vi "Find.vi"(8 "Error In":errorcluster, 10 "Key":string, 11 "Context In":refnum<class "Context.lvclass">) -> (0 "Error Out":errorcluster, 1 "Found?":bool, 2 "Datum":refnum<class "Abstract.lvclass">, 3 "Context Out":refnum<class "Context.lvclass">)   [LabVIEW 2018, in "Toolkit.lvlib" / "Data.lvlib" / "Context.lvclass"]
uses:
  Context.lvclass
  Abstract/Abstract.lvclass
  Context.lvclass/Context.ctl
  Null/Null.lvclass
  D:/Users/cfield/Code/Field R&D Services/Mustache/trunk/src/Toolkit/Data/Abstract/Abstract.lvclass
  Map/Map.lvclass
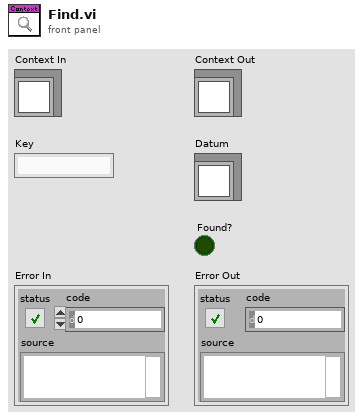
[diagram p1: front panel]
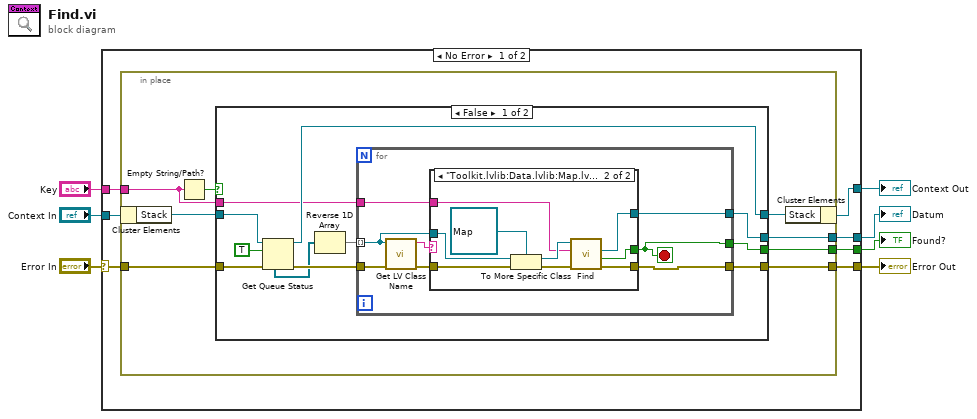
[diagram p0: block diagram]
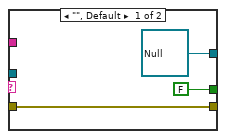
[diagram p2: hidden frame]
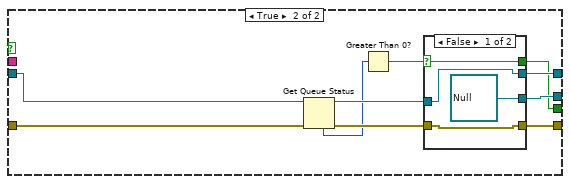
[diagram p3: hidden frame]
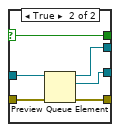
[diagram p4: hidden frame]
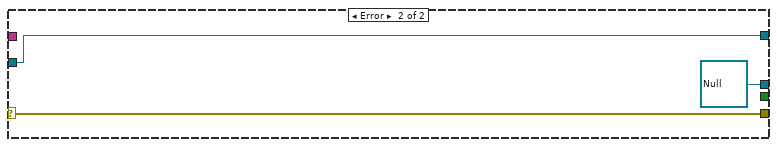
[diagram p5: hidden frame]
diagram:
  n1 = case shown="No Error" "Error In" {
    selector: "Error In" -> [w11 w75]
    tunnel: [w14 refnum<class "Null.lvclass"> refnum ("Toolkit.lvlib:Data.lvlib:Null.lvclass")] -> w7
    tunnel: [w13 w75] -> w6
    tunnel: [w12 _] -> w5
    tunnel: "Context In" -> [w10 w76]
    tunnel: [w9 w76] -> w2
    tunnel: "Key" -> [w8 _]
    frame No Error {
      n2 = in-place {
        in-place-border: [w22] -> w14
        in-place-border: [w21] -> w13
        in-place-border: [w20] -> w12
        in-place-border: w11 -> [w19]
        in-place-border: w8 -> [w16]
        n3 = in-place-cluster #1(w10) -> ("Stack"=w18:refnum<queue>)
        n4 = Empty String/Path?(string/path=w16) -> (empty?=w15:bool)
        n5 = case shown="False" w15 {
          tunnel: [w33 w62] -> w22
          tunnel: [w32 w54] -> w21
          tunnel: [w27 w55] -> w20
          tunnel: w19 -> [w26 w58]
          tunnel: w18 -> [w25 w61]
          tunnel: [w24 w63] -> w17
          tunnel: w16 -> [w23 _]
          frame False {
            n6 = Get Queue Status(queue=w25, return elements? (F)=TRUE, error in (no error)=w26) -> (queue out=w24:refnum<queue>, error out=w31:errorcluster, elements=w29:refnum<class "Abstract.lvclass">[])  [unwired: 5 out]
            n7 = Reverse 1D Array(array=w29) -> (reversed array=w30:refnum<class "Abstract.lvclass">[])
            n8 = for {
              tunnel: w30 -> [w38] mode=indexing
              tunnel: w23 -> [w37]
              tunnel: w31 -> [w41]
              tunnel: [w36] -> w32
              tunnel: [w35] -> w33
              tunnel: [w34] -> w27
              stop <- w34 stop-if-true
              n9 = call <vilib>:"Get LV Class Name.vi"("error in (no error)"=w41, "object"=w38) -> ("error out"=w39:errorcluster, "class name"=w40:string)  [unwired: 8 in]
              n10 = case shown="\"Toolkit.lvlib:Data.lvlib:Map.lvclass\"" w40 {
                tunnel: w39 -> [w43 w53]
                tunnel: w38 -> [_ w52]
                tunnel: w37 -> [_ w48]
                tunnel: [w43 w47] -> w36
                tunnel: [FALSE ("Found?") w45] -> w34
                tunnel: [refnum<class "Null.lvclass"> refnum ("Toolkit.lvlib:Data.lvlib:Null.lvclass") w46] -> w35
                frame "", Default {
                }
                frame "Toolkit.lvlib:Data.lvlib:Map.lvclass" {
                  n11 = To More Specific Class(target class=refnum<class "Map.lvclass"> refnum ("Toolkit.lvlib:Data.lvlib:Map.lvclass"), reference=w52, error in=w53) -> (specific class reference=w49:refnum<class "Map.lvclass">, error out=w50:errorcluster)
                  n12 = call "Find.vi"("Error In"=w50, "Key"=w48, "Map In"=w49) -> ("Error Out"=w47:errorcluster, "Found?"=w45:bool, "Value"=w46:refnum<class "Abstract.lvclass">)  [unwired: 5 in, 1 out]
                }
              }
            }
          }
          frame True {
            n13 = Get Queue Status(queue=w61, error in (no error)=w58) -> (queue out=w60:refnum<queue>, error out=w59:errorcluster, # elements in queue=w57:i32)  [unwired: 1 in, 5 out]
            n14 = Greater Than 0?(x=w57) -> (x > 0?=w56:bool)
            n15 = case shown="False" w56 {
              selector: w56 -> [w66 w68]
              tunnel: [w67 w73] -> w63
              tunnel: [refnum<class "Null.lvclass"> refnum ("Toolkit.lvlib:Data.lvlib:Null.lvclass") w72] -> w62
              tunnel: w60 -> [w67 w71]
              tunnel: w59 -> [w65 w70]
              tunnel: [w66 w68] -> w55
              tunnel: [w65 w69] -> w54
              frame False {
              }
              frame True {
                n16 = Preview Queue Element(queue=w71, error in (no error)=w70) -> (queue out=w73:refnum<queue>, element=w72:refnum<class "Abstract.lvclass">, error out=w69:errorcluster)  [unwired: 1 in, 1 out]
              }
            }
          }
        }
        n17 = in-place-cluster #1("Stack"=w17) -> (w9:refnum<class "Context.lvclass">)
      }
    }
    frame Error {
    }
  }
  "Datum" <- w7
  "Error Out" <- w6
  "Found?" <- w5
  "Context Out" <- w2
